vi "Instrument Handler.vi"(10 "Calibrate":bool, 11 "ADALM2000 URI":string) -> (2 "error out":errorcluster, 3 "ADALM2000 Handle":u64 caption="Instrument Handle Out")   [LabVIEW 2022 SP3]
uses:
  libm2k_lv.dll
panel:
  out "Error Out":errorcluster
  in  "error in (no error)":errorcluster
  out "Ret Code":dbl format="%#_13g"
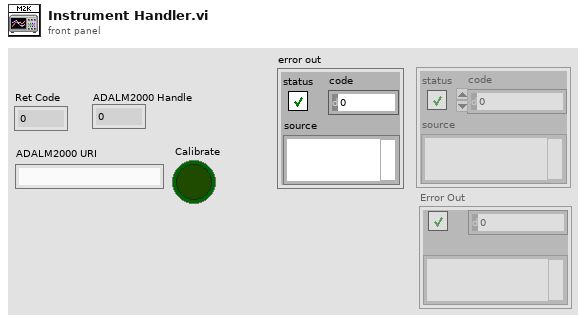
[diagram p1: front panel]
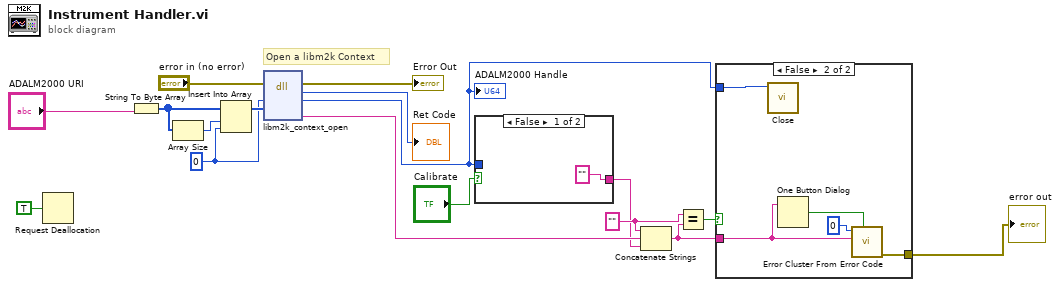
[diagram p0: block diagram]
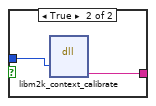
[diagram p2: hidden frame]
diagram:
  w13 = 0
  w16 = ""
  # "Open a libm2k Context"
  n1 = Request Deallocation(TRUE ("flag")) -> ()
  n2 = String To Byte Array(string="ADALM2000 URI") -> (unsigned byte array=w11:u8[])
  n3 = Array Size(array=w11) -> (size(s)=w12:i32)
  n4 = Insert Into Array(array=w11, index=w12, new element=w13) -> (w15:u8[])
  n5 = dll-call lib="libm2k_lv.*" fn="libm2k_context_open"(error in="error in (no error)", "arg1"=w13, "uri"=w15) -> (error out=→"Error Out":errorcluster, "return type"=→"Ret Code":i64, "arg1"=w3:u64, "err"=w8:string)  [unwired: 4 in, 1 out]
  "ADALM2000 Handle" <- w3
  n6 = case shown="False" "Calibrate" {
    tunnel: w3 -> [_ w20]
    tunnel: ["" w19] -> w6
    frame False {
    }
    frame True {
      n7 = dll-call lib="libm2k_lv.dll" fn="libm2k_context_calibrate"("instance"=w20) -> ("err"=w19:string)  [unwired: 6 in, 2 out]
    }
  }
  n8 = Concatenate Strings(w16, w8, w6) -> (w5:string)
  n9 = Equal?(x=w16, y=w5) -> (x = y?=w4:bool)
  n10 = case shown="False" w4 {
    tunnel: w5 -> [_ w23]
    tunnel: w3 -> [_ w22]
    tunnel: [_ w21] -> w1
    frame True {
    }
    frame False {
      n11 = call "Close.vi"("ADALM2000 Handler"=w22) -> ()  [unwired: 11 in]
      n12 = One Button Dialog(message=w23) -> (true=w25:bool)  [unwired: 1 in]
      n13 = call <vilib>:"Error Cluster From Error Code.vi"("show call chain? (False)"=w25, "error message (\"\")"=w23, "error code (0)"=0) -> ("error out"=w21:errorcluster)  [unwired: 6 in]
    }
  }
  "error out" <- w1
